vi "ATS_Busy.vi"(11 "DeviceIn":i32) -> (2 "Busy":bool, 3 "DeviceOut":i32, 5 "#Device":i32)   [LabVIEW 2015]
doc: "_____AlazarTech, Scope_____\n\nQuery the devices's busy status."
uses:
  ATS_ctl/ATS_Global_Ctrl.ctl
panel:
  out "Return Code":u32
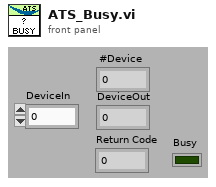
[diagram p1: front panel]
types:
  T1 = typedef "ATS_Global_Ctrl.ctl" = enum16{"Init_Device", "Clear_ALL", "Set", "Get"}
  T2 = typedef "Device_Info.ctl" = cluster{"Handle":u32, "Board":string, "CPLD":string, "MemorySize":u32, "SampleSize":u8, "ID":i32, "High_Memory":bool, "Chan/Board":u8}
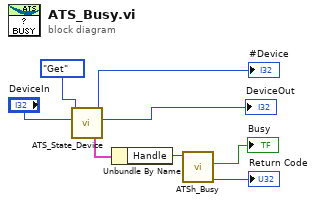
[diagram p0: block diagram]
diagram:
  n1 = call "ATS_State_Device.vi"("DeviceIn"="DeviceIn", "ATS_GBL_Ctrl"=ATS_Global_Ctrl."Get") -> ("DeviceOut"=→"DeviceOut":i32, "#Device"=→"#Device":i32, "DevInfo_Out"=w4:T2)  [unwired: 4 in, 3 out]
  n2 = Unbundle By Name(w4) -> ("Handle"=w6:u32)
  n3 = call "ATSh_Busy.vi"("Handle"=w6) -> ("Return Code"=→"Return Code":u32, "Busy"=→"Busy":bool)  [unwired: 8 in, 1 out]
